vi "SAC-Read Work.vi"(0 "path":path, 11 "Error In":errorcluster) -> (4 "Params":T1, 8 "Result":cluster{"Stimulus":dbl[], "Response":dbl[]}, 15 "error out":errorcluster)   [LabVIEW 2020]
uses:
  Typedefs/SAC-Parameters.ctl
  HRTF VIs/Typedefs/HRTF-Waveform.ctl
  HRTF VIs/Typedefs/HRTF-Window.ctl
  HRTF VIs/Typedefs/HRTF-Window Type.ctl
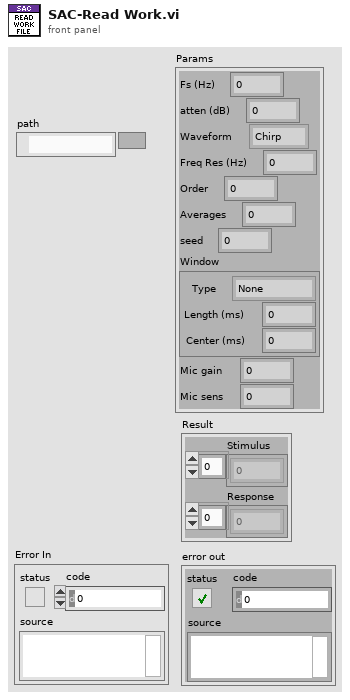
[diagram p1: front panel]
types:
  T1 = typedef "SAC-Parameters.ctl" = cluster{"Fs (Hz)":dbl, "atten (dB)":dbl, "Waveform":T2, "Freq Res (Hz)":dbl, "Order":i32, "Averages":i32, "seed":i64, "Window":T3, "Mic gain":dbl, "Mic sens":dbl}
  T2 = typedef "HRTF-Waveform.ctl" = enum16{"Chirp", "MLS"}
  T3 = typedef "HRTF-Window.ctl" = cluster{"Type":T4, "Length (ms)":dbl, "Center (ms)":dbl}
  T4 = typedef "HRTF-Window Type.ctl" = enum16{"None", "Rectangle", "Hanning"}
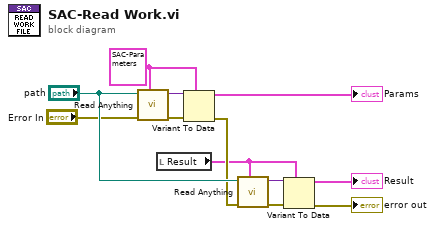
[diagram p0: block diagram]
diagram:
  w5 = T1 {"Fs (Hz)"=0.0, "atten (dB)"=0.0, "Waveform"=enum."Chirp", "Freq Res (Hz)"=0.0, "Order"=0, "Averages"=0, "seed"=-1, "Window"={"Type"=enum."None", "Length (ms)"=0.0, "Center (ms)"=0.0}, "Mic gain"=0.0, "Mic sens"=0.0} ("Params")
  n1 = call "Read Anything.vi"("Type of Anything"=w5, "Error In"="Error In", "Path (dialog)"="path") -> ("Error Out"=w3:errorcluster, "Anything"=w4:variant)  [unwired: 6 in, 1 out]
  n2 = local read "Result"() -> (w2:cluster{"Stimulus":dbl[], "Response":dbl[]})
  n3 = Variant To Data(error in=w3, type=w5, Variant=w4) -> (data=→"Params":T1, error out=w7:errorcluster)
  n4 = call "Read Anything.vi"("Type of Anything"=w2, "Error In"=w7, "Path (dialog)"="path") -> ("Error Out"=w6:errorcluster, "Anything"=w8:variant)  [unwired: 6 in, 1 out]
  n5 = Variant To Data(error in=w6, type=w2, Variant=w8) -> (data=→"Result":cluster{"Stimulus":dbl[], "Response":dbl[]}, error out=→"error out":errorcluster)
